vi "Limelight_Differential.vi"() -> (0 "DriveCommand":dbl(knob)=-0.0 scale=0.0..1.0, 1 "SteerCommand":dbl(knob)=nan scale=-1.0..1.0, 3 "TargetValid":bool)   [LabVIEW 2019]
uses:
  <vilib>/Rock Robotics/Network Tables/NT Read Number.vi
  Global Vars.vi
  <vilib>/Rock Robotics/Network Tables/NT Read Boolean.vi
panel:
  in  "x":dbl=23.05 format="%#_13g"
  out "Distance":dbl
  in  "Height":dbl=57.5
  out "Angle of Elevation":dbl
  in  "DriveDeadband":dbl
  in  "MaxDrive":dbl(slide)=0.6824817518248175 min=0.0 max=1.0 step=0.01 scale=0.0..1.0
  in  "DriveK":dbl(slide)=0.26277372262773724 min=0.0 max=1.0 step=0.05 scale=0.0..20.0
  in  "Limelight Goal Area":dbl(slide)=14.872262773722628 min=0.1 max=25.0 step=0.25 scale=0.0..1.0
  in  "AimDeadband":dbl=1.0 min=0.0 max=10.0 step=0.25
  in  "MinSteerCommand":dbl(slide)=0.40217391304347827 min=0.0 max=0.5 step=0.05 scale=0.0..0.5
  in  "SteeringK":dbl(slide)=0.025362318840579712 min=0.0 max=0.25 step=0.01 scale=0.0..0.25
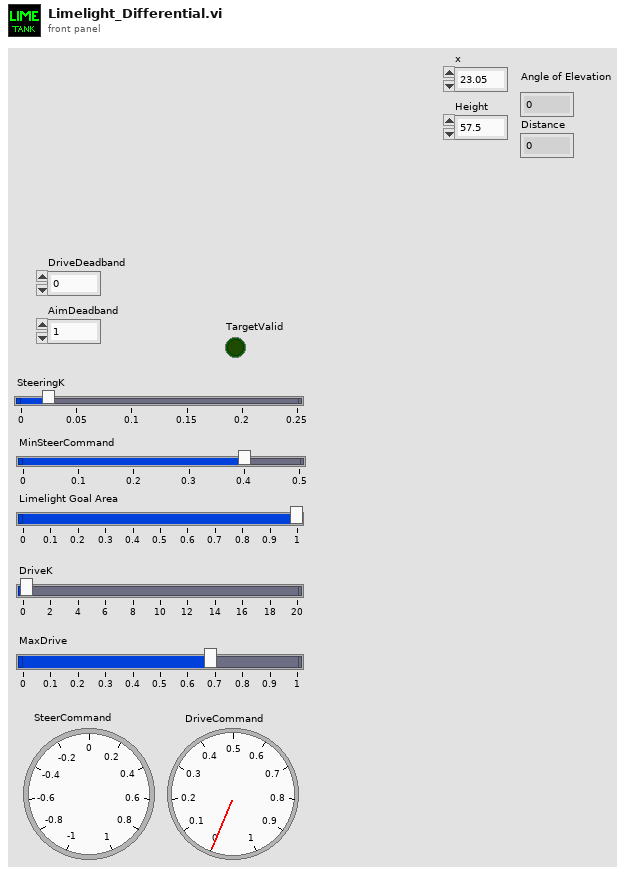
[diagram p1: front panel]
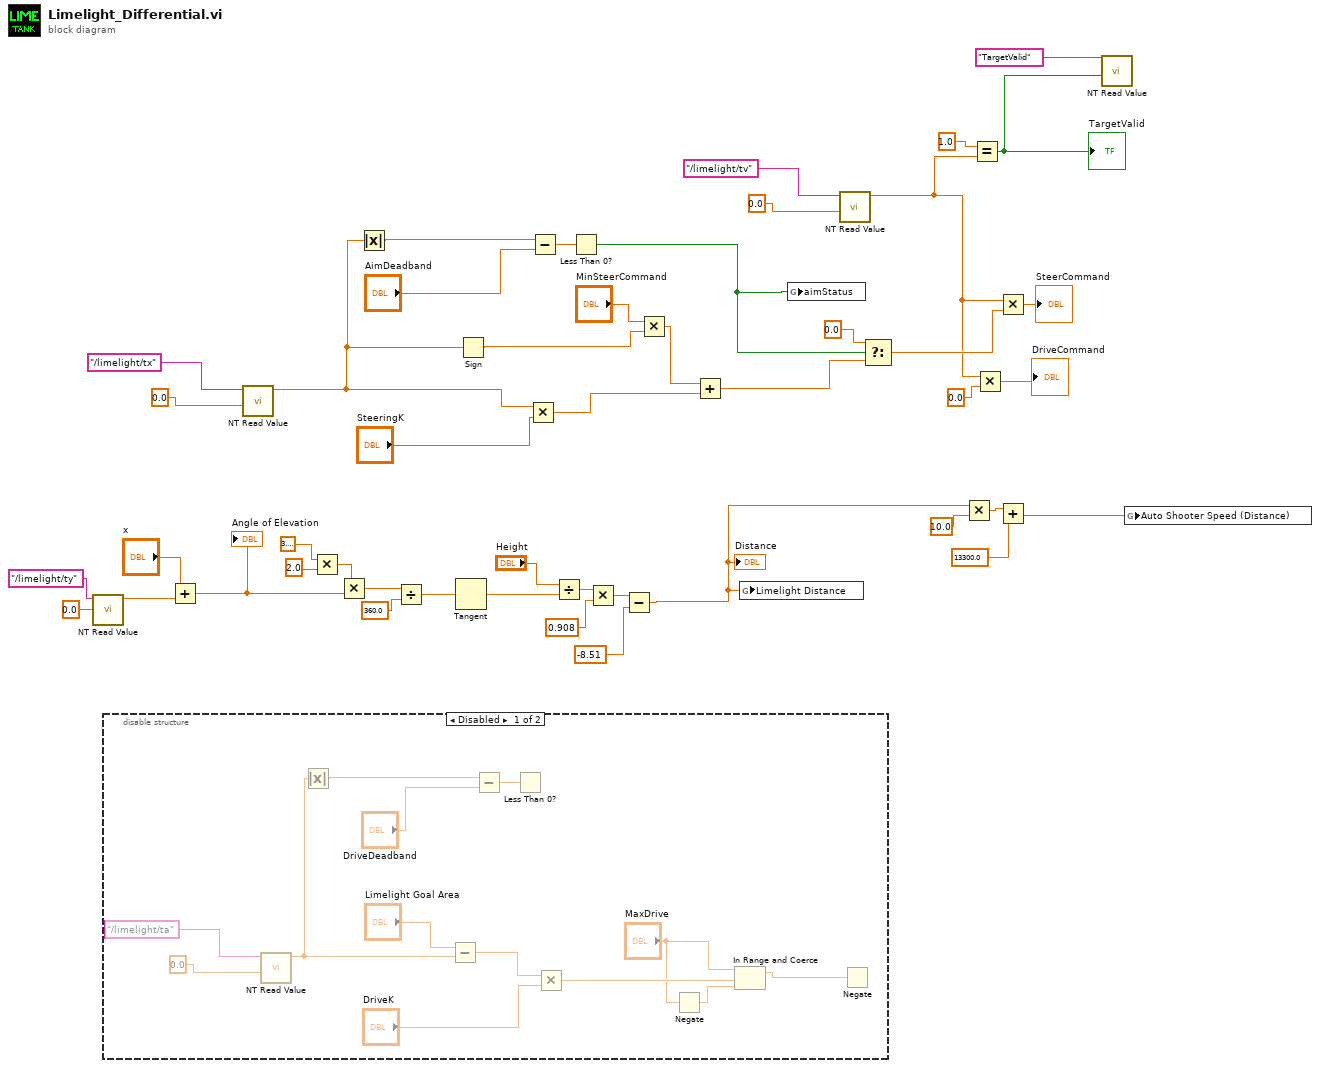
[diagram p0: block diagram]
diagram:
  n1 = call-poly <vilib>:"NT Read Value.vi"("Default Value"=0.0, "Name"="/limelight/ty") -> ("Numeric"=w16:dbl)  [unwired: 8 in, 1 out]
  n2 = disable-structure shown="Disabled" {
    frame Disabled {
      n3 = call-poly <vilib>:"NT Read Value.vi"("Default Value"=0.0, "Name"="/limelight/ta") -> ("Numeric"=w48:dbl)  [unwired: 8 in, 1 out]
      n4 = Absolute Value(x=w48) -> (abs(x)=w49:dbl)
      n5 = Subtract(x="Limelight Goal Area", y=w48) -> (x-y=w55:dbl)
      n6 = Subtract(x=w49, y="DriveDeadband") -> (x-y=w50:dbl)
      n7 = Less Than 0?(x=w50) -> ()  [unwired: 1 out]
      n8 = Multiply(x=w55, y="DriveK") -> (x*y=w54:dbl)
      n9 = Negate(x="MaxDrive") -> (-x=w51:dbl)
      n10 = In Range and Coerce(upper limit="MaxDrive", x=w54, lower limit=w51) -> (coerced(x)=w53:dbl)  [unwired: 1 out]
      n11 = Negate(x=w53) -> ()  [unwired: 1 out]
    }
    frame Enabled {
    }
  }
  n12 = Add(x="x", y=w16) -> (x+y=w15:dbl)
  "Angle of Elevation" <- w15
  n13 = call-poly <vilib>:"NT Read Value.vi"("Default Value"=0.0, "Name"="/limelight/tx") -> ("Numeric"=w30:dbl)  [unwired: 8 in, 1 out]
  n14 = Multiply(x=3.141592653589793, y=2.0) -> (x*y=w22:dbl)
  n15 = Multiply(x=w22, y=w15) -> (x*y=w21:dbl)
  n16 = Absolute Value(x=w30) -> (abs(x)=w43:dbl)
  n17 = Divide(x=w21, y=360.0) -> (x/y=w19:dbl)
  n18 = Tangent(1:w19) -> (0:w17:dbl)
  n19 = Sign(1:w30) -> (0:w32:dbl)
  n20 = Multiply(x=w30, y="SteeringK") -> (x*y=w40:dbl)
  n21 = Subtract(x=w43, y="AimDeadband") -> (x-y=w45:dbl)
  n22 = Divide(x="Height", y=w17) -> (x/y=w13:dbl)
  n23 = Less Than 0?(x=w45) -> (x < 0?=w9:bool)
  n24 = Multiply(x=w13, y=0.908) -> (x*y=w12:dbl)
  n25 = Subtract(x=w12, y=-8.51) -> (x-y=w4:dbl)
  "Distance" <- w4
  n26 = Multiply(x="MinSteerCommand", y=w32) -> (x*y=w42:dbl)
  n27 = Add(x=w42, y=w40) -> (x+y=w29:dbl)
  n28 = global write "Global Vars.vi" "Limelight Distance"(w4) -> ()
  n29 = global write "Global Vars.vi" "aimStatus"(w9) -> ()
  n30 = call-poly <vilib>:"NT Read Value.vi"("Default Value"=0.0, "Name"="/limelight/tv") -> ("Numeric"=w27:dbl)  [unwired: 8 in, 1 out]
  n31 = Select(t=0.0, s=w9, f=w29) -> (s? t:f=w35:dbl)
  n32 = Multiply(x=w4, y=10.0) -> (x*y=w7:dbl)
  n33 = Equal?(x=1.0, y=w27) -> (x = y?=w11:bool)
  "TargetValid" <- w11
  n34 = Multiply(x=w27, y=0.0) -> (x*y=→"DriveCommand":dbl)
  n35 = Multiply(x=w27, y=w35) -> (x*y=→"SteerCommand":dbl)
  n36 = Add(x=w7, y=13300.0) -> (x+y=w3:dbl)
  n37 = call-poly <vilib>:"NT Read Value.vi"("Default Value"=w11, "Name"="TargetValid") -> ()  [unwired: 8 in, 2 out]
  n38 = global write "Global Vars.vi" "Auto Shooter Speed (Distance)"(w3) -> ()
